vi "StateMachineInit.vi"(6 "ManualMotionWaveform":dbl[](array[numeric]), 7 "Enum":T2, 8 "Error In":errorcluster, 10 "FPGA.SEin":T1, 11 "FPGA.FBin":T3) -> (0 "error out":errorcluster, 2 "FPGA.SEout":T1, 3 "FPGA.FBout":T3)   [LabVIEW 2016]
uses:
  controls/FPGAVIreferenceTypeDef.ctl
  controls/EnumSM.ctl
  controls/FPGAVIreferenceTypeDefScanEngine.ctl
  controls/Enum.ctl
  controls/ScanWaveform.ctl
  <vilib>/Utility/error.llb/Error Cluster From Error Code.vi
  <vilib>/rvi/errors/niLvFpgaAdjustHostInterfaceError.vi
  <vilib>/rvi/interface/nirviReadWriteControl/nirviReadWriteControl.xnode
  FPGA Bitfiles/qnmController797_usbRIO_controllerFPGAmu.lvbitx
  NiFpgaLv.dll
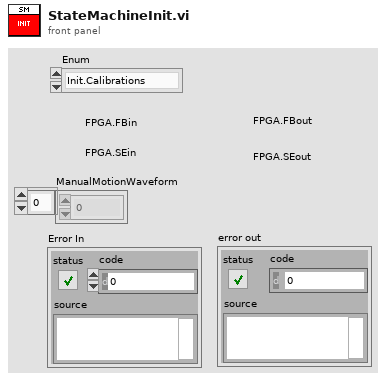
[diagram p1: front panel]
types:
  T1 = typedef "FPGAVIreferenceTypeDefScanEngine.ctl" = refnum<k20>
  T2 = typedef "EnumSM.ctl" = enum16{"Init.Calibrations", "Init.Excitation", "Init.StepMotor", "Init.FeedbackMotion", "Init.Scan", "Init.Signals", "Init.System", "Init.Waveform", "Init.ZController", "Send.Waveform", "Correct.Hysteresis"}
  T3 = typedef "FPGAVIreferenceTypeDef.ctl" = refnum<k20>
  T4 = typedef "Enum.ctl" = enum16{"Init", "Read", "Write"}
  T5 = cluster{"slowMoveWavePts":u16, "slowMoveAccelPts":u16, "moveSpeedSec":dbl}
  T6 = cluster{"write":bool, "Address":i8, "Data":bool[]}
  T7 = cluster{"write":bool, "Address":i8, "Data":bool[]}[]
  T8 = cluster{"write":bool, "data":fxp<+,16,1>, "index":u16}
  T9 = typedef "ScanWaveform.ctl" = enum16{"Sine", "Triangle", "Rounded"}
  T10 = cluster{"slowWavePts":u16, "fastWavePts":u16, "slowWaveType":T9, "fastWaveType":T9, "slowRoundPts":u16, "fastRoundPts":u16, "singleDirectionScan":bool}
  T11 = cluster{"enableManualMotion":bool, "doMove":bool, "integratorTarget":fxp<+/-,22,2>, "clocks":cluster{"inverseDecimation":fxp<+,22,0>, "decimation":u16, "waveSize":u16, "pixelDecimation":u16}}
  T12 = cluster{"upperLimit":fxp<+/-,28,4>, "lowerLimit":fxp<+/-,28,4>}
  T13 = cluster{"write":bool, "index":u16, "data":fxp<+/-,18,5>}
  T14 = typedef "ScanParametersAllTypeDef.ctl" = cluster{"fastRoundPts":u16, "slowRoundPts":u16, "fastWaveType":T9, "slowWaveType":T9, "fastWavePts":u16, "slowWavePts":u16, "outputRateHz":u32, "yOffset":dbl, "xOffset":dbl, "scanSizeSlow":dbl, "scanSizeFast":dbl, "rotation":dbl, "timePerLine":dbl, "numLines":u16, "pointsPerLine":u32, "scanEnable":bool, "slowMoveWavePts":u16, "slowMoveAccelPts":u16, "moveSpeedSec":dbl, "singleDirectionScan":bool}
  T15 = cluster{"Width":dbl, "Height":dbl, "X Offset":dbl, "Y Offset":dbl, "Angle":dbl, "Pixels/Line":u16, "Lines":u16, "Time/Line":dbl, "Scan Rate":dbl}
  T16 = cluster{"startFwd":u16, "endFwd":u16, "startBwd":u16, "endBwd":u16, "disableBlanking":bool, "useFineCounter":bool}
  T17 = cluster{"Waveform Shape Fast In":dbl[], "Waveform Shape Slow In":dbl[]}
  T18 = cluster{"outputRate":u16, "fastDecFactor":u16, "outWaveSizeFast":u16, "pplUpsampling":u16, "numLines":u16, "se.p.fastInvDec":fxp<+,22,0>, "se.p.slowUpStep":fxp<+,28,0>, "se.p.outWaveSizeSlow":u16, "blankingMax":u32, "se.p.fastBlanking":cluster{"startFwd":u32, "endFwd":u32, "startBwd":u32, "endBwd":u32, "disableBlanking":bool, "useCoarseCounter":bool}}
  T19 = cluster{"liftHeight":fxp<+/-,15,4>, "disengagePos":fxp<+/-,22,1>}
  T20 = cluster{"CorrectionToFGV":bool, "PolynomCoeff":dbl[], "CorrectionToFPGA":bool}
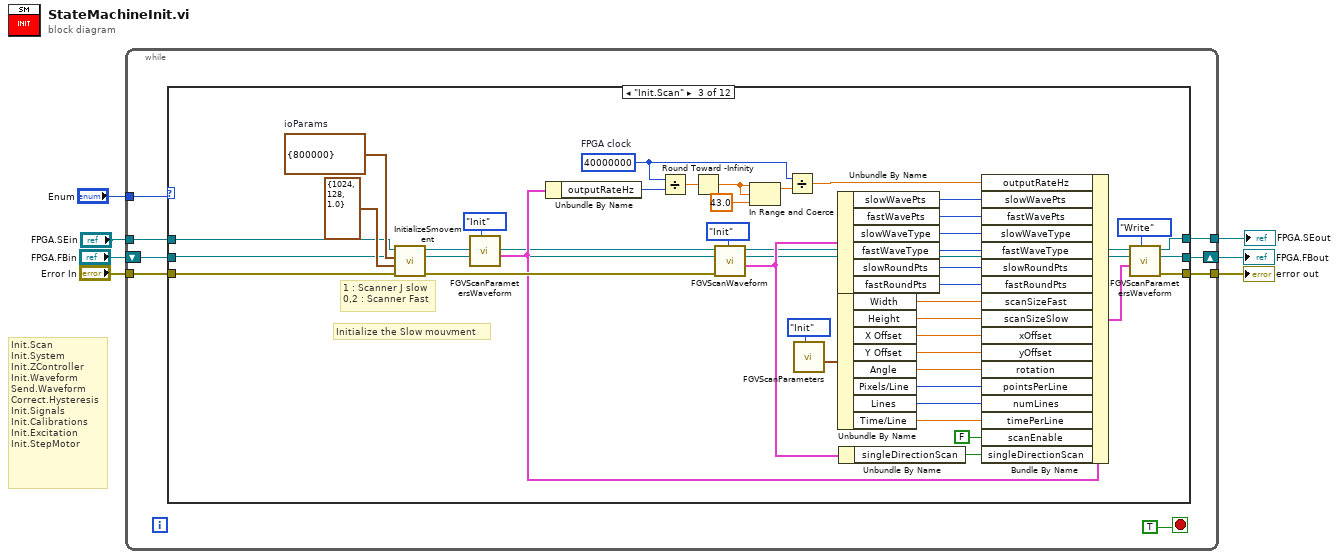
[diagram p0: block diagram]
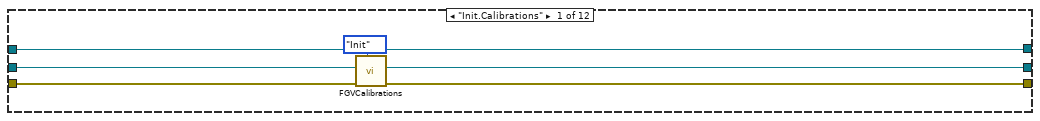
[diagram p2: hidden frame]
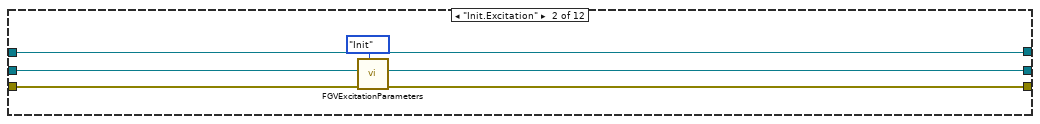
[diagram p3: hidden frame]
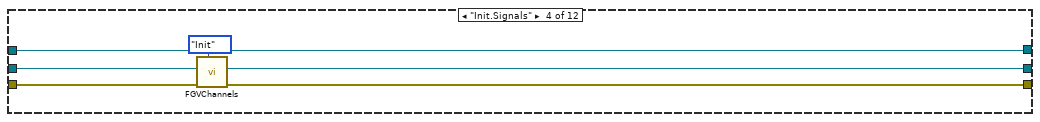
[diagram p4: hidden frame]
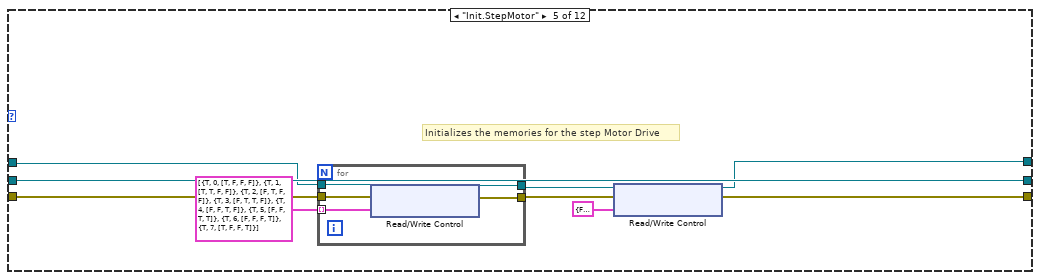
[diagram p5: hidden frame]
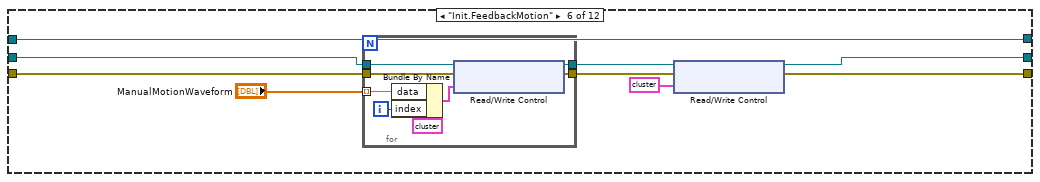
[diagram p6: hidden frame]
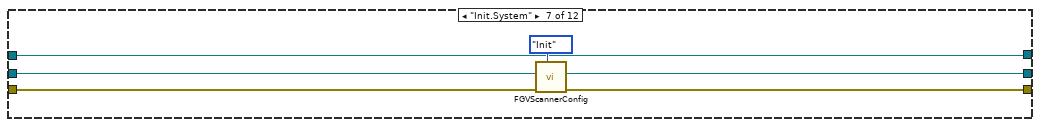
[diagram p7: hidden frame]
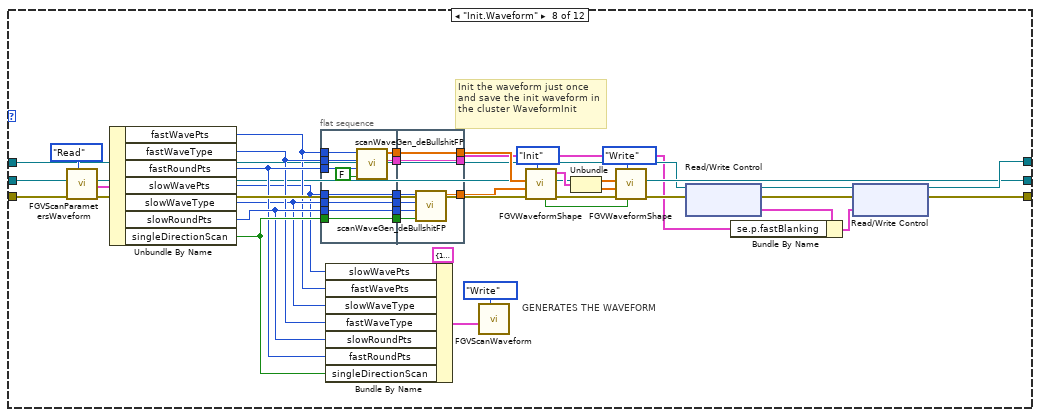
[diagram p8: hidden frame]
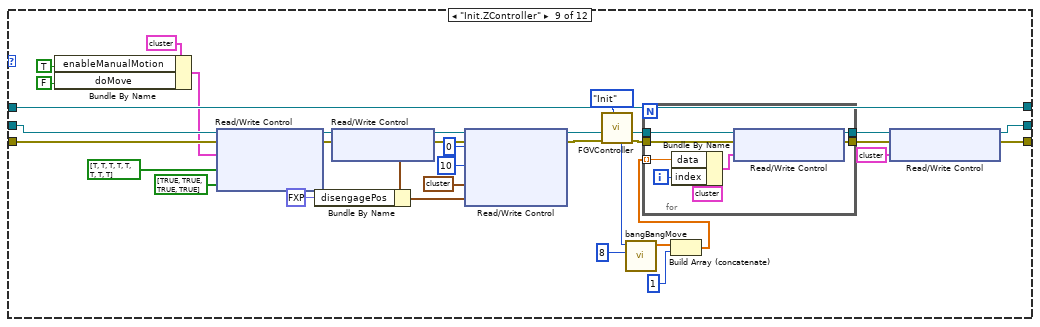
[diagram p9: hidden frame]
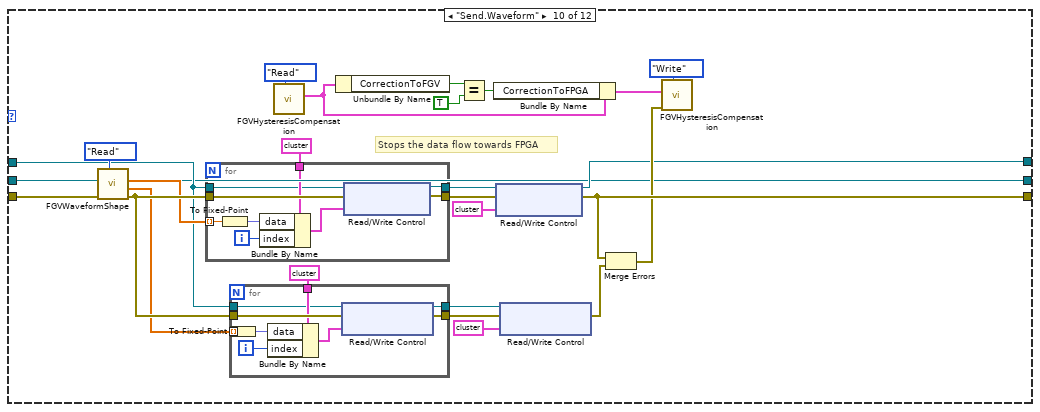
[diagram p10: hidden frame]
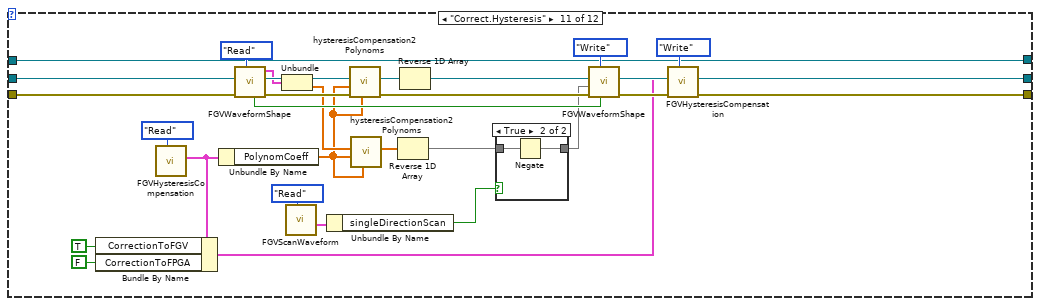
[diagram p11: hidden frame]
diagram:
  # "Init.Scan\nInit.System\nInit.ZController\nInit.Waveform\nSend.Waveform\nCorrect.Hysteresis\nInit.Signals\nInit.Calibrations\nInit.Excitation\nInit.StepMotor"
  n1 = while {
    shift-right: [w13] -> w5
    shift-left: "FPGA.FBin" -> [w15]
    tunnel: "Error In" -> [w14]
    tunnel: [w12] -> w4
    tunnel: "FPGA.SEin" -> [w10]
    tunnel: [w9] -> w1
    tunnel: "Enum" -> [w8]
    stop <- TRUE stop-if-true
    n2 = case shown="\"Init.Scan\"" w8 {
      tunnel: w15 -> [w17 w25 w26 w66 w78 w86 w105 w113 w194 w203 w274 w280]
      tunnel: w14 -> [w19 w24 w61 w68 w73 w85 w104 w116 w193 w216 w249 w279]
      tunnel: [w17 w25 w26 w66 w78 w88 w105 w113 w171 w203 w274 w280] -> w13
      tunnel: [w18 w23 w29 w67 w72 w87 w103 w115 w170 w208 w248 w279] -> w12
      tunnel: w10 -> [w16 w21 w28 w65 w71 w92 w101 w111 w167 w205 w247 w278]
      tunnel: [w16 w21 w27 w65 w70 w92 w101 w114 w167 w204 w247 w278] -> w9
      frame "Init.Calibrations" {
        n3 = call "FGVCalibrations.vi"("Enum"=Enum."Init", "error in"=w19) -> ("error out"=w18:errorcluster)  [unwired: 8 in, 1 out]
      }
      frame "Init.Excitation" {
        n4 = call "FGVExcitationParameters.vi"("Enum"=Enum."Init", "error in"=w24) -> ("error out"=w23:errorcluster)  [unwired: 5 in, 4 out]
      }
      frame "Init.Scan" {
        w31 = u32 40000000  # FPGA clock
        w62 = cluster{"outputRateHz":u32} {"outputRateHz"=800000}  # ioParams
        # "1 : Scanner J slow\n0,2 : Scanner Fast"
        # "Initialize the Slow mouvment"
        n5 = call "InitializeSmovement.vi"("error in"=w61, "slowMoveParams"=T5 {"slowMoveWavePts"=1024, "slowMoveAccelPts"=128, "moveSpeedSec"=1.0}, "ioParams"=w62, "FPGAInterfaceIn"=w28) -> ("error out"=w64:errorcluster, "FPGAInterfaceOut"=w27:T1)  [unwired: 6 in]
        n6 = call "FGVScanParametersWaveform.vi"("Enum"=Enum."Init") -> ("Parameters Out"=w35:T14)  [unwired: 9 in, 1 out]
        n7 = Unbundle By Name(w35) -> ("outputRateHz"=w36:u32)
        n8 = Divide(x=w31, y=w36) -> (x/y=w40:dbl)
        n9 = Round Toward -Infinity(1:w40) -> (0:w41:dbl)
        n10 = call "FGVScanWaveform.vi"("Enum"=Enum."Init", "error in"=w64) -> ("scanWaveFormCtl Out"=w30:T10)  [unwired: 8 in, 1 out]
        n11 = In Range and Coerce(upper limit=w41, x=w41, lower limit=43.0) -> (coerced(x)=w38:dbl)  [unwired: 1 out]
        n12 = Divide(x=w31, y=w38) -> (x/y=w37:dbl)
        n13 = call "FGVScanParameters.vi"("Enum"=Enum."Init") -> ("Scan Parameters Out"=w32:T15)  [unwired: 9 in, 1 out]
        n14 = Unbundle By Name(w30) -> ("slowWavePts"=w47:u16, "fastWavePts"=w46:u16, "slowWaveType"=w45:T9, "fastWaveType"=w44:T9, "slowRoundPts"=w43:u16, "fastRoundPts"=w42:u16)
        n15 = Unbundle By Name(w32) -> ("Width"=w54:dbl, "Height"=w53:dbl, "X Offset"=w52:dbl, "Y Offset"=w51:dbl, "Angle"=w50:dbl, "Pixels/Line"=w34:u16, "Lines"=w33:u16, "Time/Line"=w49:dbl)
        n16 = Unbundle By Name(w30) -> ("singleDirectionScan"=w60:bool)
        n17 = Bundle By Name(cluster=w35, "outputRateHz"=w37, "slowWavePts"=w47, "fastWavePts"=w46, "slowWaveType"=w45, "fastWaveType"=w44, "slowRoundPts"=w43, "fastRoundPts"=w42, "scanSizeFast"=w54, "scanSizeSlow"=w53, "xOffset"=w52, "yOffset"=w51, "rotation"=w50, "pointsPerLine"=w34, "numLines"=w33, "timePerLine"=w49, "scanEnable"=FALSE, "singleDirectionScan"=w60) -> (w58:T14)
        n18 = call "FGVScanParametersWaveform.vi"("Enum"=Enum."Write", "Parameters In"=w58) -> ("error out"=w29:errorcluster)  [unwired: 8 in, 1 out]
      }
      frame "Init.Signals" {
        n19 = call "FGVChannels.vi"("Enum"=Enum."Init", "error in"=w68) -> ("error out"=w67:errorcluster)  [unwired: 5 in, 4 out]
      }
      frame "Init.StepMotor" {
        # "Initializes the memories for the step Motor Drive"
        n20 = for {
          tunnel: T7 [{"write"=TRUE, "Address"=0, "Data"=[TRUE, FALSE, FALSE, FALSE]}, {"write"=TRUE, "Address"=1, "Data"=[TRUE, TRUE, FALSE, FALSE]}, {"write"=TRUE, "Address"=2, "Data"=[FALSE, TRUE, FALSE, FALSE]}, {"write"=TRUE, "Address"=3, "Data"=[FALSE, TRUE, TRUE, FALSE]}, {"write"=TRUE, "Address"=4, "Data"=[FALSE, FALSE, TRUE, FALSE]}, {"write"=TRUE, "Address"=5, "Data"=[FALSE, FALSE, TRUE, TRUE]}, {"write"=TRUE, "Address"=6, "Data"=[FALSE, FALSE, FALSE, TRUE]}, {"write"=TRUE, "Address"=7, "Data"=[TRUE, FALSE, FALSE, TRUE]}] ("Array") -> [w82] mode=indexing
          tunnel: w71 -> [w80]
          tunnel: [w83] -> w76
          tunnel: w73 -> [w79]
          tunnel: [w81] -> w77
          n21 = xnode "Read/Write Control"("FPGA VI Reference In"=w80, "error in"=w79, "smd.p.writeMem"=w82) -> ("FPGA VI Reference Out"=w83:T1, "error out"=w81:errorcluster)
        }
        n22 = xnode "Read/Write Control"("FPGA VI Reference In"=w76, "error in"=w77, "smd.p.writeMem"=T6 {"write"=FALSE, "Address"=0, "Data"=[TRUE, FALSE, FALSE, FALSE]} ("halfStepWrite 2")) -> ("FPGA VI Reference Out"=w70:T1, "error out"=w72:errorcluster)
      }
      frame "Init.FeedbackMotion" {
        n23 = for {
          tunnel: w86 -> [w98]
          tunnel: [w97] -> w90
          tunnel: w85 -> [w100]
          tunnel: [w99] -> w91
          tunnel: "ManualMotionWaveform" -> [w93] mode=indexing
          i -> [w94]
          n24 = Bundle By Name(cluster=T8 {"write"=TRUE, "data"=0.0, "index"=0} ("fb.mot.m.motion"), "data"=w93, "index"=w94) -> (w96:T8)
          n25 = xnode "Read/Write Control"("FPGA VI Reference In"=w98, "error in"=w100, "fb.mot.m.motion"=w96) -> ("FPGA VI Reference Out"=w97:T3, "error out"=w99:errorcluster)
        }
        n26 = xnode "Read/Write Control"("FPGA VI Reference In"=w90, "error in"=w91, "fb.mot.m.motion"=T8 {"write"=FALSE, "data"=0.0, "index"=0}) -> ("FPGA VI Reference Out"=w88:T3, "error out"=w87:errorcluster)
      }
      frame "Init.System" {
        n27 = call "FGVScannerConfig.vi"("Enum"=Enum."Init", "error in"=w104) -> ("error out"=w103:errorcluster)  [unwired: 7 in, 2 out]
      }
      frame "Init.Waveform" {
        # "GENERATES THE WAVEFORM"
        # "Init the waveform just once\nand save the init waveform in the cluster WaveformInit"
        n28 = call "FGVScanParametersWaveform.vi"("Enum"=Enum."Read", "error in"=w116) -> ("error out"=w144:errorcluster, "Parameters Out"=w134:T14)  [unwired: 8 in]
        n29 = Unbundle By Name(w134) -> ("fastWavePts"=w120:u16, "fastWaveType"=w122:T9, "fastRoundPts"=w123:u16, "slowWavePts"=w119:u16, "slowWaveType"=w121:T9, "slowRoundPts"=w124:u16, "singleDirectionScan"=w125:bool)
        n30 = flat-sequence {
          tunnel: w120 -> [w154]
          tunnel: w122 -> [w153]
          tunnel: w123 -> [w152]
          tunnel: [w150] -> w141
          tunnel: w119 -> [w150]
          tunnel: w121 -> [w149]
          tunnel: [w149] -> w140
          tunnel: [w148] -> w139
          tunnel: w124 -> [w148]
          tunnel: w125 -> [w147]
          tunnel: [w147] -> w138
          tunnel: [w146] -> w137
          tunnel: [w145] -> w136
          tunnel: w141 -> [w161]
          tunnel: w140 -> [w160]
          tunnel: w139 -> [w159]
          tunnel: w138 -> [w158]
          tunnel: w137 -> [w157]
          tunnel: [w157] -> w133
          tunnel: [w156] -> w142
          tunnel: w136 -> [w155]
          tunnel: [w155] -> w108
          frame #0 {
            n31 = call "scanWaveGen_deBullshitFP.vi"("singleDirScan"=FALSE, "numRoundingPts"=w152, "scanWaveForm"=w153, "numPts"=w154) -> ("blankingParams"=w145:T16, "outWave"=w146:dbl[])  [unwired: 6 in]
          }
          frame #1 {
            n32 = call "scanWaveGen_deBullshitFP.vi"("singleDirScan"=w158, "numRoundingPts"=w159, "scanWaveForm"=w160, "numPts"=w161) -> ("outWave"=w156:dbl[])  [unwired: 6 in, 1 out]
          }
        }
        n33 = Bundle By Name(cluster=T10 {"slowWavePts"=1024, "fastWavePts"=1024, "slowWaveType"=enum."Triangle", "fastWaveType"=enum."Rounded", "slowRoundPts"=8, "fastRoundPts"=32, "singleDirectionScan"=TRUE} ("scanWaveFormCtl In"), "slowWavePts"=w119, "fastWavePts"=w120, "slowWaveType"=w121, "fastWaveType"=w122, "slowRoundPts"=w124, "fastRoundPts"=w123, "singleDirectionScan"=w125) -> (w126:T10)
        n34 = call "FGVScanWaveform.vi"("Enum"=Enum."Write", "scanWaveFormCtl In"=w126) -> ()  [unwired: 8 in, 2 out]
        n35 = call "FGVWaveformShape.vi"("Enum"=Enum."Init", "error in"=w144, "Waveform Shape Slow In"=w142, "Waveform Shape Fast In"=w133) -> ("error out"=w143:errorcluster, "WaveformInit"=w130:T17, "Framing up? (down: f) out"=w117:bool)  [unwired: 3 in, 2 out]
        n36 = Unbundle(w130) -> ("Waveform Shape Fast In"=w129:dbl[], "Waveform Shape Slow In"=w128:dbl[])
        n37 = call "FGVWaveformShape.vi"("Framing up? (down: f) In"=w117, "Enum"=Enum."Write", "error in"=w143, "Waveform Shape Slow In"=w128, "Waveform Shape Fast In"=w129) -> ("error out"=w110:errorcluster)  [unwired: 2 in, 4 out]
        n38 = xnode "Read/Write Control"("FPGA VI Reference In"=w111, "error in"=w110) -> ("FPGA VI Reference Out"=w112:T1, "error out"=w109:errorcluster, "se.p.clocks"=w107:T18)
        n39 = Bundle By Name(cluster=w107, "se.p.fastBlanking"=w108) -> (w106:T18)
        n40 = xnode "Read/Write Control"("FPGA VI Reference In"=w112, "error in"=w109, "se.p.clocks"=w106) -> ("FPGA VI Reference Out"=w114:T1, "error out"=w115:errorcluster)
      }
      frame "Init.ZController" {
        n41 = Bundle By Name(cluster=T11 {"enableManualMotion"=FALSE, "doMove"=FALSE, "integratorTarget"=0.0, "clocks"={"inverseDecimation"=0.0, "decimation"=0, "waveSize"=0, "pixelDecimation"=0}} ("fb.mot.p.params"), "enableManualMotion"=TRUE, "doMove"=FALSE) -> (w163:T11)
        n42 = xnode "Read/Write Control"("FPGA VI Reference In"=w194, "error in"=w193, "fb.mot.p.params"=w163, "flt.bypass1"=bool[] [TRUE, TRUE, TRUE, TRUE, TRUE, TRUE, TRUE, TRUE] ("sosBypass"), "flt.bypass2"=bool[] [TRUE, TRUE, TRUE, TRUE]) -> ("FPGA VI Reference Out"=w182:T3, "error out"=w181:errorcluster)
        n43 = xnode "Read/Write Control"("FPGA VI Reference In"=w182, "error in"=w181) -> ("FPGA VI Reference Out"=w184:T3, "error out"=w188:errorcluster, "fb.loff.p.params"=w186:T19)
        n44 = Bundle By Name(cluster=w186, "disengagePos"=fxp<+/-,22,1> -1.0) -> (w185:T19)
        n45 = xnode "Read/Write Control"("FPGA VI Reference In"=w184, "error in"=w188, "fb.i.source"=u8 0, "ort.p.waveSize"=u16 10, "fb.p.limits"=T12 {"upperLimit"=1.0, "lowerLimit"=-1.0}, "fb.loff.p.params"=w185) -> ("FPGA VI Reference Out"=w169:T3, "error out"=w180:errorcluster)
        n46 = call "FGVController.vi"("Enum"=Enum."Init", "error in"=w180) -> ("error out"=w168:errorcluster, "moveWaveSizeOut"=w175:u16)  [unwired: 5 in, 3 out]
        n47 = call "bangBangMove.vi"("numRoundingPts"=u16 8, "numPts"=w175) -> ("roundedHalfTriangle"=w177:dbl[])  [unwired: 9 in]
        n48 = Build Array (concatenate)(w177, u16 1 ("numRoundingPts")) -> (w166:dbl[])
        n49 = for {
          tunnel: w169 -> [w200]
          tunnel: [w199] -> w173
          tunnel: w168 -> [w202]
          tunnel: [w201] -> w174
          tunnel: w166 -> [w195] mode=indexing
          i -> [w196]
          n50 = Bundle By Name(cluster=T8 {"write"=TRUE, "data"=0.0, "index"=0} ("fb.mot.m.motion"), "data"=w195, "index"=w196) -> (w198:T8)
          n51 = xnode "Read/Write Control"("FPGA VI Reference In"=w200, "error in"=w202, "fb.mot.m.motion"=w198) -> ("FPGA VI Reference Out"=w199:T3, "error out"=w201:errorcluster)
        }
        n52 = xnode "Read/Write Control"("FPGA VI Reference In"=w173, "error in"=w174, "fb.mot.m.motion"=T8 {"write"=FALSE, "data"=0.0, "index"=0}) -> ("FPGA VI Reference Out"=w171:T3, "error out"=w170:errorcluster)
      }
      frame "Send.Waveform" {
        # "Stops the data flow towards FPGA"
        n53 = call "FGVWaveformShape.vi"("Enum"=Enum."Read", "error in"=w216) -> ("error out"=w228:errorcluster, "Waveform Shape Slow Out"=w219:dbl[], "Waveform Shape Fast Out"=w223:dbl[])  [unwired: 5 in, 2 out]
        n54 = for {
          tunnel: w223 -> [w243] mode=indexing
          tunnel: T13 {"write"=TRUE, "index"=0, "data"=0.0} ("slowWaveWrite") -> [w242]
          tunnel: w205 -> [w241]
          tunnel: [w245] -> w225
          tunnel: w228 -> [w246]
          tunnel: [w244] -> w224
          i -> [w238]
          n55 = To Fixed-Point(number=w243) -> (fixed-point=w239:fxp<+/-,18,5>)  [unwired: 1 in]
          n56 = Bundle By Name(cluster=w242, "data"=w239, "index"=w238) -> (w240:T13)
          n57 = xnode "Read/Write Control"("FPGA VI Reference In"=w241, "error in"=w246, "se.m.fastAxis"=w240) -> ("FPGA VI Reference Out"=w245:T1, "error out"=w244:errorcluster)
        }
        n58 = for {
          tunnel: w219 -> [w234] mode=indexing
          tunnel: T13 {"write"=TRUE, "index"=0, "data"=0.0} ("slowWaveWrite") -> [w233]
          tunnel: w228 -> [w237]
          tunnel: [w235] -> w220
          tunnel: w205 -> [w232]
          tunnel: [w236] -> w221
          i -> [w229]
          n59 = To Fixed-Point(number=w234) -> (fixed-point=w230:fxp<+/-,18,5>)  [unwired: 1 in]
          n60 = Bundle By Name(cluster=w233, "data"=w230, "index"=w229) -> (w231:T13)
          n61 = xnode "Read/Write Control"("FPGA VI Reference In"=w232, "error in"=w237, "se.m.slowAxis"=w231) -> ("FPGA VI Reference Out"=w236:T1, "error out"=w235:errorcluster)
        }
        n62 = call "FGVHysteresisCompensation.vi"("Enum"=Enum."Read") -> ("HysteresisFastOut"=w209:T20)  [unwired: 8 in, 2 out]
        n63 = Unbundle By Name(w209) -> ("CorrectionToFGV"=w212:bool)
        n64 = Equal?(x=w212, y=TRUE) -> (x = y?=w215:bool)
        n65 = Bundle By Name(cluster=w209, "CorrectionToFPGA"=w215) -> (w214:T20)
        n66 = xnode "Read/Write Control"("FPGA VI Reference In"=w225, "error in"=w224, "se.m.fastAxis"=T13 {"write"=FALSE, "index"=0, "data"=0.0} ("fastWaveWrite")) -> ("FPGA VI Reference Out"=w204:T1, "error out"=w208:errorcluster)
        n67 = xnode "Read/Write Control"("FPGA VI Reference In"=w221, "error in"=w220, "se.m.slowAxis"=T13 {"write"=FALSE, "index"=0, "data"=0.0} ("fastWaveWrite")) -> ("error out"=w207:errorcluster)  [unwired: 1 out]
        n68 = Merge Errors(w208, w207) -> (w206:errorcluster)
        n69 = call "FGVHysteresisCompensation.vi"("Enum"=Enum."Write", "error in"=w206, "HysteresisFastIn"=w214) -> ()  [unwired: 6 in, 3 out]
      }
      frame "Correct.Hysteresis" {
        n70 = call "FGVHysteresisCompensation.vi"("Enum"=Enum."Read") -> ("HysteresisFastOut"=w256:T20)  [unwired: 8 in, 2 out]
        n71 = Bundle By Name(cluster=w256, "CorrectionToFGV"=TRUE ("Correction?"), "CorrectionToFPGA"=FALSE) -> (w257:T20)
        n72 = Unbundle By Name(w256) -> ("PolynomCoeff"=w259:dbl[])
        n73 = call "FGVWaveformShape.vi"("Enum"=Enum."Read", "error in"=w249) -> ("error out"=w264:errorcluster, "WaveformInit"=w265:T17, "Framing up? (down: f) out"=w267:bool)  [unwired: 5 in, 2 out]
        n74 = Unbundle(w265) -> ("Waveform Shape Fast In"=w269:dbl[], "Waveform Shape Slow In"=w263:dbl[])
        n75 = call "FGVScanWaveform.vi"("Enum"=Enum."Read") -> ("scanWaveFormCtl Out"=w252:T10)  [unwired: 9 in, 1 out]
        n76 = Unbundle By Name(w252) -> ("singleDirectionScan"=w250:bool)
        n77 = call "hysteresisCompensation2Polynoms.vi"("PolynomBWD"=w259, "error in (no error)"=w264, "PolynomFWD"=w259, "Uncorrected Shape"=w269) -> ("error out"=w272:errorcluster, "Corrected Shape"=w268:dbl[])  [unwired: 6 in]
        n78 = call "hysteresisCompensation2Polynoms.vi"("PolynomBWD"=w259, "PolynomFWD"=w259, "Uncorrected Shape"=w263) -> ("Corrected Shape"=w262:dbl[])  [unwired: 7 in, 1 out]
        n79 = Reverse 1D Array(array=w262) -> (reversed array=w251:dbl[])
        n80 = Reverse 1D Array(array=w268) -> (reversed array=w270:dbl[])
        n81 = case shown="True" w250 {
          tunnel: [w275 w277] -> w261
          tunnel: w251 -> [w275 w276]
          frame False {
          }
          frame True {
            n82 = Negate(x=w276) -> (-x=w277:dbl[])
          }
        }
        n83 = call "FGVWaveformShape.vi"("Framing up? (down: f) In"=w267, "Enum"=Enum."Write", "error in"=w272, "Waveform Shape Slow In"=w261, "Waveform Shape Fast In"=w270) -> ("error out"=w273:errorcluster)  [unwired: 2 in, 4 out]
        n84 = call "FGVHysteresisCompensation.vi"("Enum"=Enum."Write", "error in"=w273, "HysteresisFastIn"=w257) -> ("error out"=w248:errorcluster)  [unwired: 6 in, 2 out]
      }
      frame Default {
      }
    }
  }
  "FPGA.FBout" <- w5
  "error out" <- w4
  "FPGA.SEout" <- w1
